vi "Get settings chain.vi"(8 "error in (no error)":errorcluster, 11 "CascadeBase in":refnum<class "Cascade.lvclass">) -> (0 "error out":errorcluster, 1 "class name":string[](array[string]), 2 "settings":variant[](array[variant]), 3 "CascadeBase out":refnum<class "Cascade.lvclass">)   [LabVIEW 2012, in "Cascade.lvclass"]
doc: "Returns an array of variants containing the settings clusters of each class in the inheritance chain (lowest child class first), together with an array of all class names in the inheritance chain.\n\nFor classes without settings cluster, the settings chain contains empty variants."
uses:
  Cascade.lvclass
  <vilib>/Distrio/Murmex/Murmex/Murmex.lvclass
  Cascade.lvclass/Cascade.ctl
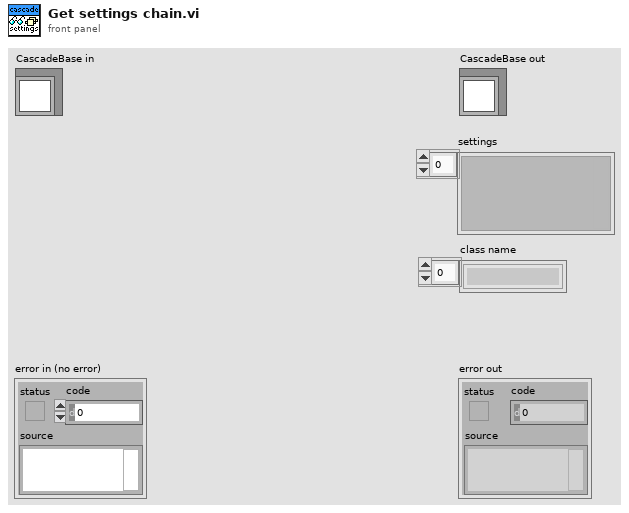
[diagram p1: front panel]
types:
  T1 = typedef "Cascade.lvclass/settings.ctl" = cluster{"Gain":dbl, "Exposure":dbl[unit], "Path":path, "filename":string, "PID gains":cluster{"proportional gain (Kc)":dbl, "integral time (Ti, min)":dbl, "derivative time (Td, min)":dbl}}
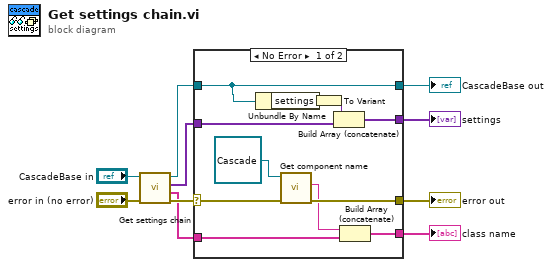
[diagram p0: block diagram]
diagram:
  n1 = call-parent "Get settings chain.vi"("error in (no error)"="error in (no error)", "MurmexBase in"="CascadeBase in") -> ("error out"=w3:errorcluster, "class name"=w2:string[], "settings"=w4:variant[], "MurmexBase out"=w7:refnum<class "Cascade.lvclass">)  [unwired: 6 in]
  n2 = case shown="No Error" w3 {
    selector: w3 -> [w21 w22]
    tunnel: [w20 w22] -> w8
    tunnel: w7 -> [w15 w23]
    tunnel: [w15 w23] -> w6
    tunnel: [w16 _] -> w5
    tunnel: w4 -> [w14 _]
    tunnel: w2 -> [w13 _]
    tunnel: [w11 _] -> w1
    frame No Error {
      n3 = Unbundle By Name(w15) -> ("settings"=w17:T1)
      n4 = call <vilib>:"Get component name.vi"("error in (no error)"=w21, "Murmex in"=refnum<class "Cascade.lvclass"> refnum ("Cascade.lvclass")) -> ("error out"=w20:errorcluster, "component name"=w12:string)  [unwired: 7 in, 1 out]
      n5 = To Variant(anything=w17) -> (Variant=w18:variant)
      n6 = Build Array (concatenate)(w18, w14) -> (w16:variant[])
      n7 = Build Array (concatenate)(w12, w13) -> (w11:string[])
    }
    frame Error {
    }
  }
  "error out" <- w8
  "CascadeBase out" <- w6
  "settings" <- w5
  "class name" <- w1
